vi "Get Active Button.vi"(8 "error in (no error)":errorcluster, 11 "QMenu Class in":refnum<class "QMenu Class.lvclass">) -> (0 "error out":errorcluster, 2 "Active Event Data":T1, 3 "QMenu Class out":refnum<class "QMenu Class.lvclass">)   [LabVIEW 2020, in "QTab.lvlib" / "QMenu Class.lvclass"]
uses:
  QMenu Class.lvclass
  Active Event Data.ctl
  Command.ctl
  QMenu Class.lvclass/QMenu Class.ctl
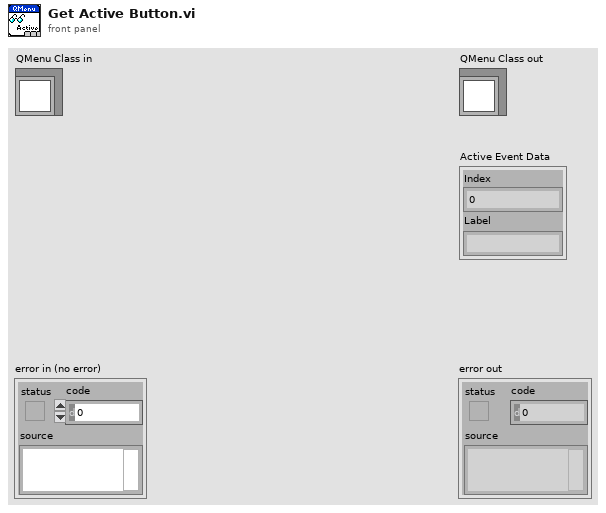
[diagram p1: front panel]
types:
  T1 = typedef "QTab.lvlib/QMenu Class.lvclass/Active Event Data.ctl" = cluster{"Index":i32, "Label":string}
  T2 = typedef "QTab.lvlib/QMenu Class.lvclass/Command.ctl" = enum16{"Initialize", "Get Active Button", "Set Active Button", "Set Button Attribute", "Add Button", "Close Button", "Draw", "Stop"}
  T3 = typedef "QTab.lvlib/QMenu Class.lvclass/Button Attribute.ctl" = cluster{"Label":string, "Button Text":string, "Closable":bool, "Draggable":bool}
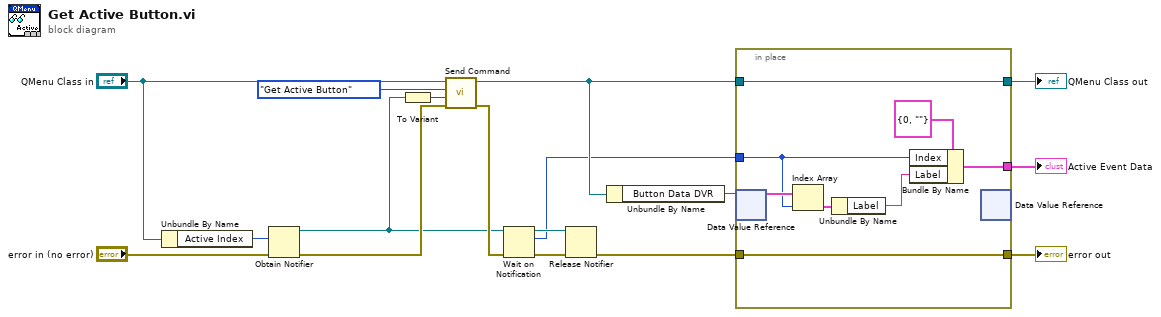
[diagram p0: block diagram]
diagram:
  n1 = Unbundle By Name("QMenu Class in") -> ("Active Index"=w8:i32)
  n2 = Obtain Notifier(notification data type=w8, error in (no error)="error in (no error)") -> (notifier out=w12:refnum<notifier>, error out=w15:errorcluster)  [unwired: 2 in, 1 out]
  n3 = To Variant(anything=w12) -> (Variant=w14:variant)
  n4 = call "Send Command.vi"("error in (no error)"=w15, "Data"=w14, "Command"=Command."Get Active Button", "QMenu Class in"="QMenu Class in") -> ("error out"=w13:errorcluster, "QMenu Class out"=w5:refnum<class "QMenu Class.lvclass">)  [unwired: 6 in]
  n5 = Wait on Notification(notifier=w12, error in (no error)=w13) -> (notifier out=w11:refnum<notifier>, notification=w3:i32, error out=w10:errorcluster)  [unwired: 2 in, 1 out]
  n6 = Release Notifier(notifier=w11, error in (no error)=w10) -> (error out=w6:errorcluster)  [unwired: 1 in, 2 out]
  n7 = Unbundle By Name(w5) -> ("Button Data DVR"=w7:refnum<data-value>)
  n8 = in-place {
    in-place-border: w6 -> [w23]
    in-place-border: w5 -> [w25]
    in-place-border: [w25] -> w4
    in-place-border: w3 -> [w20]
    in-place-border: [w23] -> w2
    in-place-border: [w18] -> w1
    n9 = in-place-dvr #1(w7) -> (w24:T3[])  [unwired: 1 out]
    n10 = Index Array(array=w24, index=w20) -> (element=w22:T3)
    n11 = Unbundle By Name(w22) -> ("Label"=w19:string)
    n12 = Bundle By Name(cluster=T1 {"Index"=0, "Label"=""} ("Active Event Data"), "Index"=w20, "Label"=w19) -> (w18:T1)
    n13 = in-place-dvr #1() -> ()  [unwired: 1 in, 2 out]
  }
  "error out" <- w2
  "QMenu Class out" <- w4
  "Active Event Data" <- w1
